vi "planarIrregularFF.vi"(4 "ForceDesired":dbl, 5 "FMFF":dbl[](array[numeric]), 6 "BoundsY":dbl[](array[numeric]), 7 "Bounds X":dbl[](array[numeric]), 8 "Center":dbl[](array[numeric]), 9 "ViconData":dbl[](array[numeric])) -> (2 "ActiveFF":bool, 3 "DesiredFM_FF":dbl[](array[numeric]))   [LabVIEW 2017]
uses:
  <vilib>/Analysis/_algsub.llb/Real Vector Norm.vi
  <vilib>/imath/engines/lvmath2/RunTimeEngine/Managers/WorkSpace/UID Generator.vi
  <vilib>/imath/engines/lvmath2/RunTimeEngine/BuiltInFunctions/is_inpolygon/NIMS_is_inpolygon(V).vi
  <vilib>/imath/engines/lvmath2/RunTimeEngine/RunTimeType/NIMS_RunTimeType_From StrictType (excl LVString).vi
  <instcachedir>/0/NIMS_RunTimeType_From StrictType (excl LVString)_1019F277F0A747EDBCA0F6C52CA54500.lvgen/NIMS_RunTimeType_From StrictType (excl LVString)_1019F277F0A747EDBCA0F6C52CA54500_000.vi
  <vilib>/imath/engines/lvmath2/RunTimeEngine/RunTimeType/NIMS_RunTimeType_Set Source Original Bool.vi
  <vilib>/imath/engines/lvmath2/RunTimeEngine/ErrorHandling/NIMS_Error From Error Code.vi
  <vilib>/imath/engines/lvmath2/RunTimeEngine/LocalVariableDefStatement/MC_LocalVariableDefStatement_Display.vi
  <vilib>/imath/engines/lvmath2/RunTimeEngine/Managers/SymbolTable/Clear UID.vi
  <vilib>/imath/engines/lvmath2/RunTimeEngine/NodeEndStatement/NIMS_NodeEndStatement_Output.vi
  <instcachedir>/0/NIMS_NodeEndStatement_Output_53EC0D466D134D7ABD903AC30B43404B.lvgen/NIMS_NodeEndStatement_Output_53EC0D466D134D7ABD903AC30B43404B_012.vi
  <vilib>/imath/engines/lvmath2/RunTimeEngine/ErrorHandling/NIMS_Finalize Error.vi
  <vilib>/Analysis/NI_AALPro.lvlib
  <vilib>/imath/engines/lvmath2/RunTimeEngine/Managers/SymbolTable/NIMS_WorkSpace.lvlib
panel:
  out "Current_point":dbl[](array[numeric])
  out "center position":dbl[](array[numeric])
  # "Irregular Force Field"
  # "INPUTS"
  # "Irregular FF Boundary Pts"
  # "OUTPUTS:"
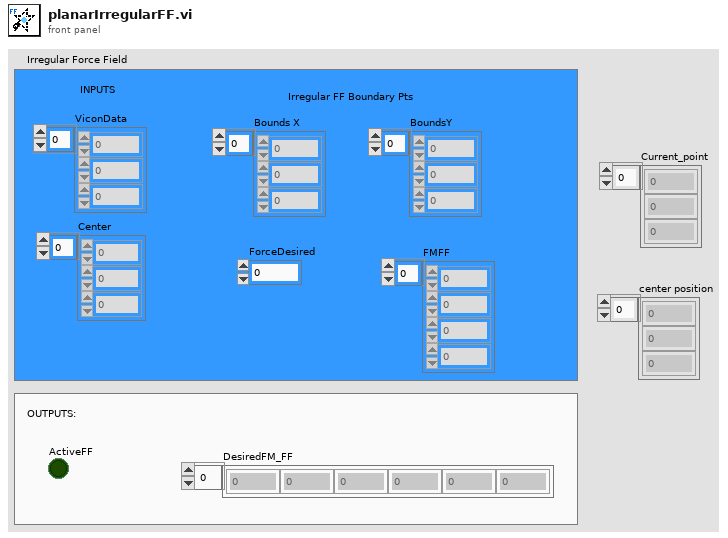
[diagram p1: front panel]
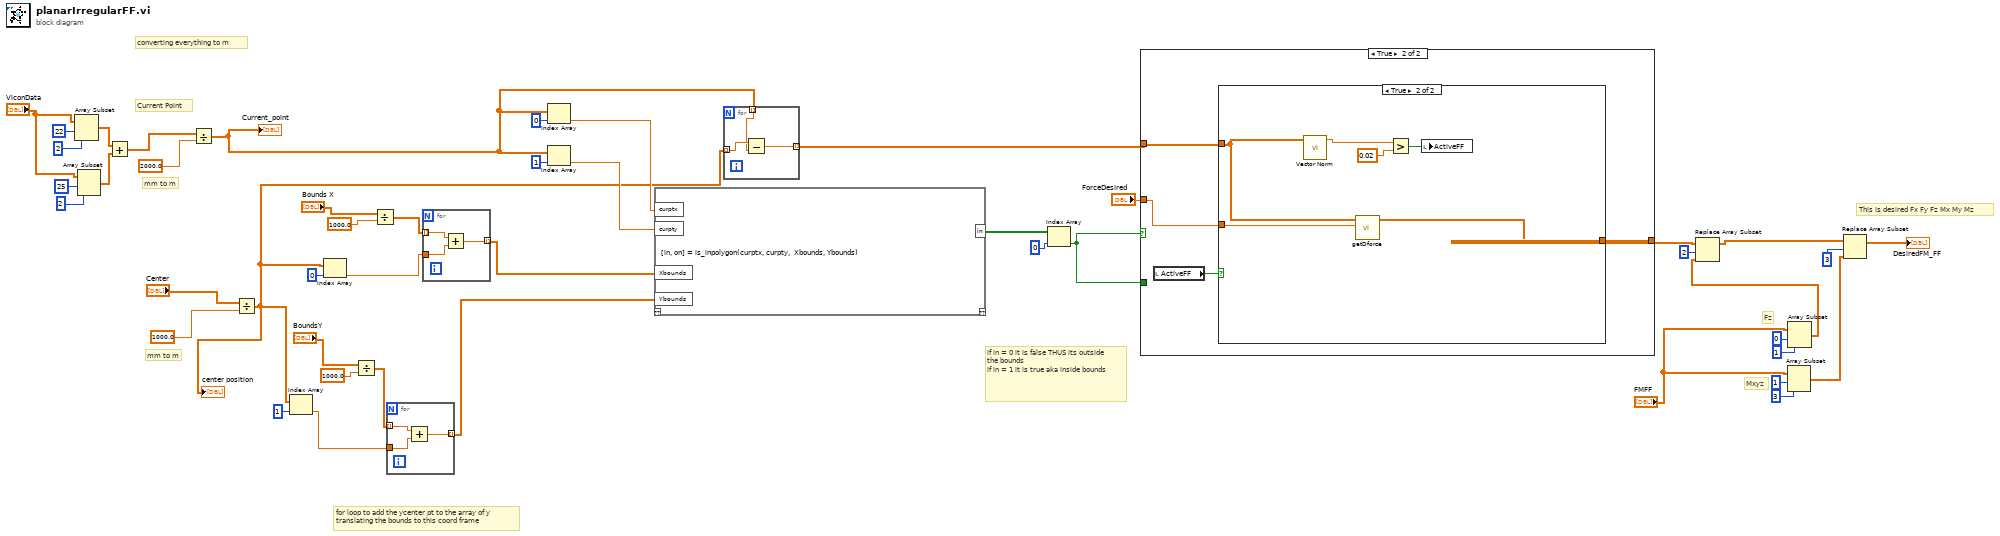
[diagram p0: block diagram]
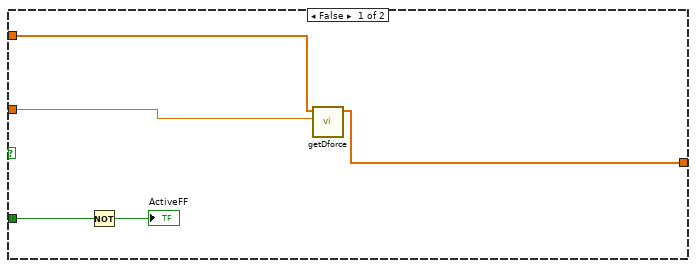
[diagram p2: hidden frame]
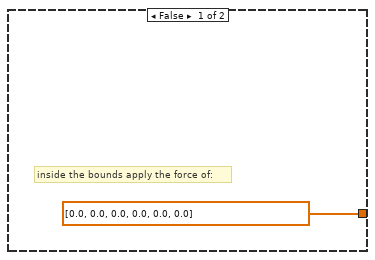
[diagram p3: hidden frame]
diagram:
  # "Current Point"
  # "mm to m"
  # "for loop to add the ycenter pt to the array of y\ntranslating the bounds to this coord frame"
  # "This is desired Fx Fy Fz Mx My Mz"
  # "converting everything to m"
  # "Fz"
  # "Mxyz"
  # "if in = 0 it is false THUS its outside the bounds\nif in = 1 it is true aka inside bounds"
  # "mm to m"
  n1 = Array Subset(array="ViconData", index=22, length=2) -> (w7:dbl[])
  n2 = Array Subset(array="ViconData", index=25, length=2) -> (w6:dbl[])
  n3 = Add(x=w7, y=w6) -> (x+y=w5:dbl[])
  n4 = Divide(x=w5, y=2000.0) -> (x/y=w4:dbl[])
  "Current_point" <- w4
  n5 = Divide(x="Center", y=1000.0) -> (x/y=w18:dbl[])
  "center position" <- w18
  n6 = Index Array(array=w18, index=1) -> (element=w29:dbl)
  n7 = Index Array(array=w18, index=0) -> (element=w25:dbl)
  n8 = Divide(x="BoundsY", y=1000.0) -> (x/y=w28:dbl[])
  n9 = Divide(x="Bounds X", y=1000.0) -> (x/y=w24:dbl[])
  n10 = for {
    tunnel: w29 -> [w49]
    tunnel: w28 -> [w48] mode=indexing
    tunnel: [w47] -> w27 mode=indexing
    n11 = Add(x=w48, y=w49) -> (x+y=w47:dbl)
  }
  n12 = for {
    tunnel: w25 -> [w52]
    tunnel: w24 -> [w51] mode=indexing
    tunnel: [w50] -> w23 mode=indexing
    n13 = Add(x=w51, y=w52) -> (x+y=w50:dbl)
  }
  n14 = Index Array(array=w4, index=0) -> (element=w21:dbl)
  n15 = Index Array(array=w4, index=1) -> (element=w19:dbl)
  n16 = mathscript code="[in, on] = is_inpolygon(curptx, curpty,  Xbounds, Ybounds)"("Xbounds"=w23, "Ybounds"=w27, "curptx"=w21, "curpty"=w19) -> ("in"=w45:bool[])  [unwired: 1 in, 1 out]
  n17 = for {
    tunnel: w18 -> [w54] mode=indexing
    tunnel: w4 -> [w53] mode=indexing
    tunnel: [w55] -> w17 mode=indexing
    n18 = Subtract(x=w54, y=w53) -> (x-y=w55:dbl)
  }
  n19 = Index Array(array=w45, index=0) -> (element=w2:bool)
  n20 = case shown="True" w2 {
    tunnel: [w58 w64] -> w33
    tunnel: w17 -> [w60 w62]
    tunnel: "ForceDesired" -> [w59 w61]
    tunnel: w2 -> [w57 _]
    frame False {
      n21 = Not(x=w57) -> (.not. x?=→"ActiveFF":bool)
      n22 = call "getDforce.vi"("ForceDesired"=w59, "Desired Direction"=w60) -> ("FX FY 0 0 0 0"=w58:dbl[])  [unwired: 5 in]
    }
    frame True {
      n23 = local read "ActiveFF"() -> (w63:bool)
      n24 = case shown="True" w63 {
        tunnel: [dbl[] [0.0, 0.0, 0.0, 0.0, 0.0, 0.0] w71] -> w64
        tunnel: w62 -> [_ w66]
        tunnel: w61 -> [_ w67]
        frame False {
          # "inside the bounds apply the force of:"
        }
        frame True {
          n25 = call-poly <vilib>:"Vector Norm.vi"("Input Vector"=w66) -> ("norm"=w70:dbl)  [unwired: 9 in, 1 out]
          n26 = call "getDforce.vi"("ForceDesired"=w67, "Desired Direction"=w66) -> ("FX FY 0 0 0 0"=w71:dbl[])  [unwired: 5 in]
          n27 = Greater?(x=w70, y=0.02) -> (0:w68:bool)
          n28 = local write "ActiveFF"(w68) -> ()
        }
      }
    }
  }
  n29 = Array Subset(array="FMFF", index=1, length=3) -> (w35:dbl[])
  n30 = Array Subset(array="FMFF", index=0, length=1) -> (w34:dbl[])
  n31 = Replace Array Subset(array=w33, new element=w34, index=2) -> (w41:dbl[])
  n32 = Replace Array Subset(array=w41, new element=w35, index=3) -> (→"DesiredFM_FF":dbl[])
